vi "Read Data.vi"(0 "TCP Socket in":refnum<class "Socket Communication.lvclass">, 2 "bytes":i32=128, 5 "error in (no error)":errorcluster) -> (14 "TCP Socket out":refnum<class "Socket Communication.lvclass">, 15 "data":string, 19 "error out":errorcluster)   [LabVIEW 2016, in "Socket Communication.lvclass"]
uses:
  Socket Communication.lvclass
  Socket Communication.lvclass/Socket Communication.ctl
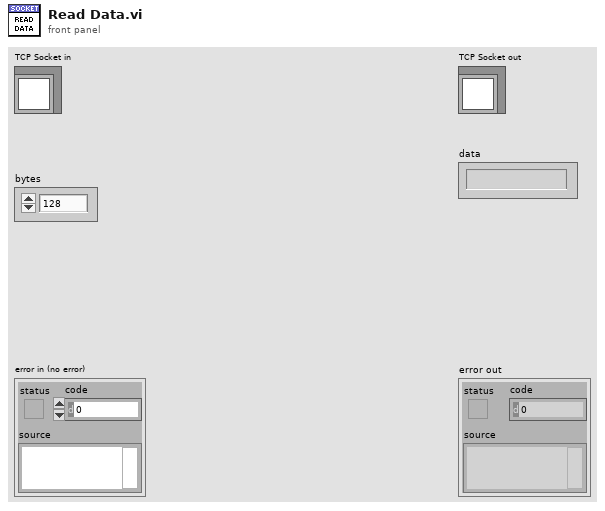
[diagram p1: front panel]
types:
  T1 = enum16{"Standard", "Buffered", "CRLF", "Immediate"}
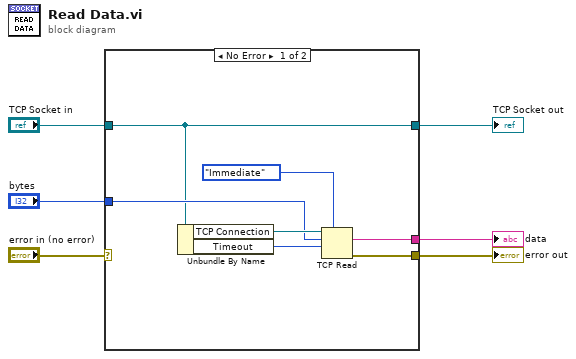
[diagram p0: block diagram]
diagram:
  n1 = case shown="No Error" "error in (no error)" {
    selector: "error in (no error)" -> [_ w15]
    tunnel: [w11 w15] -> w5
    tunnel: [w8 w14] -> w3
    tunnel: "TCP Socket in" -> [w8 w14]
    tunnel: [w10 _] -> w2
    tunnel: "bytes" -> [w9 _]
    frame No Error {
      n2 = Unbundle By Name(w8) -> ("TCP Connection"=w12:refnum<k5>, "Timeout"=w7:i32)
      n3 = TCP Read(connection ID=w12, bytes to read=w9, 7:T1."Immediate" ("mode (standard)"), 9:w7) -> (data out=w10:string, error out=w11:errorcluster)  [unwired: 1 in, 1 out]
    }
    frame Error {
    }
  }
  "error out" <- w5
  "TCP Socket out" <- w3
  "data" <- w2
